vi "Get Hist.vi"() -> ()   [LabVIEW 2018]
doc: "Get Hist: This example is to obtain a histogram example, which is a tool for visualizing the distribution of image pixel values. A histogram displays the frequency or quantity of each pixel value in an image, which can help analyze the contrast, brightness, and color information of the image."
uses:
  vi.lib/VIRobotics/opencv_yiku/Mat/Mat_8U/Mat_8U.lvclass
  D:/Program Files/company/National Instruments/LabVIEW 2018/vi.lib/addons/VIRobotics/opencv_yiku/Mat/Mat/Mat.lvclass
  vi.lib/VIRobotics/opencv_yiku/Cap/Cap.lvclass
  vi.lib/VIRobotics/opencv_yiku/opencv_yiku.lvlib
  vi.lib/VIRobotics/opencv_yiku/Mat/Mat/Mat.lvclass
panel:
  out "Waveform Graph":sgl[][](graph)
  in  "stop":bool
  out "src pic":picture
  # "Overview: Demonstrates how to get hist.\nRequirements: Windows.\nInstructions: \n1.Run the VI"
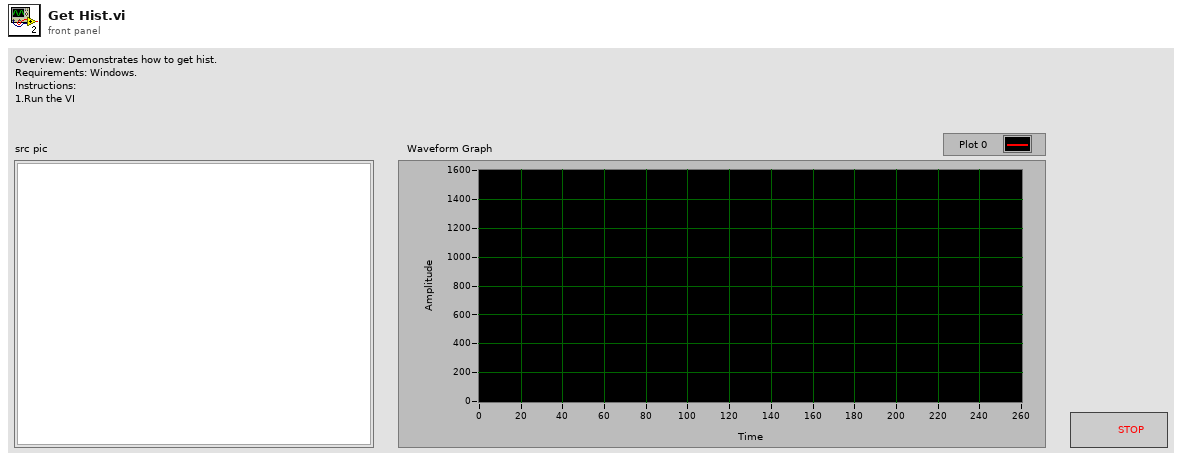
[diagram p1: front panel]
types:
  T1 = enum16{"COLOR_BGR2BGRA", "COLOR_BGRA2BGR", "COLOR_BGR2RGBA", "COLOR_RGBA2BGR", "COLOR_BGR2RGB", "COLOR_BGRA2RGBA", "COLOR_BGR2GRAY", "COLOR_RGB2GRAY", "COLOR_GRAY2BGR", "COLOR_GRAY2BGRA"}
  T2 = typedef "imagedata.ctl" = cluster{"image type":i32, "image depth":i32, "image":u8[], "mask":u8[], "colors":u32[], "Rectangle":cluster{"left":i16, "top":i16, "right":i16, "bottom":i16}}
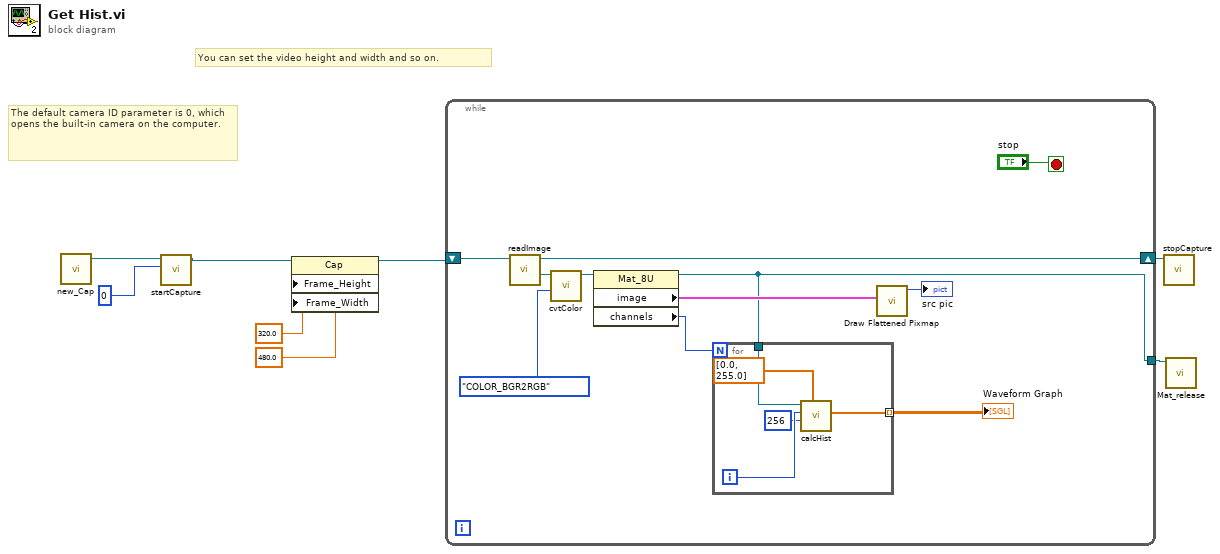
[diagram p0: block diagram]
diagram:
  # "You can set the video height and width and so on."
  # "The default camera ID parameter is 0, which opens the built-in camera on the computer."
  n1 = call "new_Cap.vi"() -> ("Cap out"=w8:refnum<class "Cap.lvclass">)  [unwired: 10 in, 1 out]
  n2 = call "startCapture.vi"("cameraID"=0, "Cap in"=w8) -> ("Cap out"=w2:refnum<class "Cap.lvclass">)  [unwired: 8 in, 1 out]
  n3 = property class="Cap"(reference=w2, "Frame_Height"=320.0, "Frame_Width"=480.0) -> (reference out=w1:refnum<class "Cap.lvclass">)  [unwired: 1 in, 1 out]
  n4 = while {
    shift-right: [w18] -> w6
    shift-left: w1 -> [w19]
    tunnel: [w9] -> w5
    stop <- "stop" stop-if-true
    n5 = call "readImage.vi"("Cap in"=w19) -> ("Mat out"=w15:refnum<class "Mat_8U.lvclass">, "Cap out"=w18:refnum<class "Cap.lvclass">)  [unwired: 8 in, 1 out]
    n6 = call "cvtColor.vi"("dstCn"=T1."COLOR_BGR2RGB", "src"=w15) -> ("src out"=w14:refnum<class "Mat_8U.lvclass">)  [unwired: 7 in, 2 out]
    n7 = property class="Mat_8U"(reference=w14) -> (reference out=w9:refnum<class "Mat_8U.lvclass">, "image"=w13:T2, "channels"=w11:i32)  [unwired: 1 in, 1 out]
    n8 = for {
      N: w11 -> [_]
      tunnel: w9 -> [w24]
      tunnel: [w20] -> w10 mode=indexing
      i -> [w23]
      n9 = call "calcHist.vi"("range"=sgl[] [0.0, 255.0], "histsize"=256, "channel"=w23, "Mat in"=w24) -> ("hist"=w20:sgl[])  [unwired: 5 in, 2 out]
    }
    "Waveform Graph" <- w10
    n10 = call <vilib>:"Draw Flattened Pixmap.vi"("image data"=w13) -> ("new picture"=→"src pic":picture)  [unwired: 8 in]
  }
  n11 = call "stopCapture.vi"("Cap in"=w6) -> ()  [unwired: 10 in, 1 out]
  n12 = call "Mat_release.vi"("Mat in"=w5) -> ()  [unwired: 10 in, 1 out]
